vi "Gamma Noise.vi"(7 "initialize?":bool=TRUE, 9 "seed":i32=-1, 10 "order":i32=1, 11 "samples":i32=128) -> (0 "error":i32, 3 "gamma noise":dbl[](array[numeric]))   [LabVIEW 2020, in "NI_AALBase.lvlib"]
doc: "Generates a pseudorandom pattern of values that are the waiting times to the <B>order</B> number event of a unit mean Poisson process."
uses:
  <vilib>/Analysis/NI_AALBase.lvlib
  <resource>/lvanlys.dll
panel:
  # "Gamma Noise"
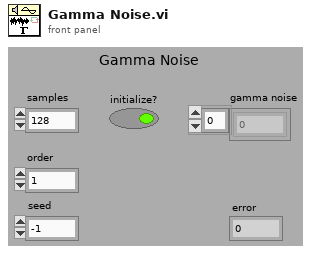
[diagram p1: front panel]
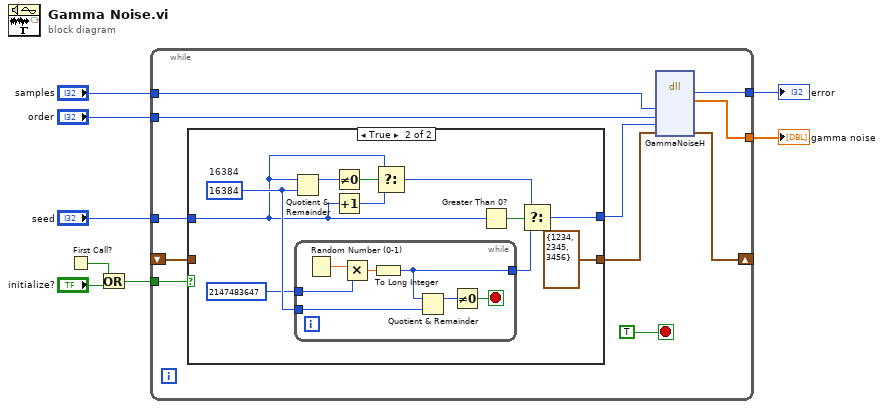
[diagram p0: block diagram]
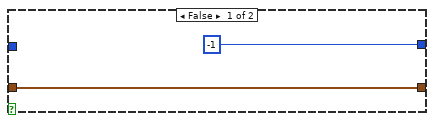
[diagram p2: hidden frame]
diagram:
  n1 = First Call?() -> (First Call?: T/F=w3:bool)
  n2 = Or(x=w3, y="initialize?") -> (x .or. y?=w1:bool)
  n3 = while {
    tunnel: [w16] -> w8
    tunnel: "seed" -> [w15]
    tunnel: "order" -> [w19]
    tunnel: "samples" -> [w18]
    shift-right: [w11] -> _
    shift-left: _ -> [w13]
    tunnel: w1 -> [w10]
    tunnel: [w9] -> w4
    stop <- TRUE stop-if-true
    n4 = case shown="True" w10 {
      tunnel: w13 -> [w21 _]
      tunnel: [w21 cluster{"xSeed":i32, "ySeed":i32, "zSeed":i32} {"xSeed"=1234, "ySeed"=2345, "zSeed"=3456} ("RNGState")] -> w12
      tunnel: [-1 ("seed") w22] -> w14
      tunnel: w15 -> [_ w23]
      frame False {
      }
      frame True {
        w25 = 16384  # 16384
        n5 = Quotient & Remainder(x=w23, y=w25) -> (x-y*floor(x/y)=w30:i32)  [unwired: 1 out]
        n6 = while {
          tunnel: [w37] -> w26
          tunnel: w25 -> [w36]
          tunnel: 2147483647 ("x") -> [w33]
          stop <- w34 stop-if-true
          n7 = Random Number (0-1)() -> (number: 0 to 1=w38:dbl)
          n8 = Multiply(x=w38, y=w33) -> (x*y=w39:dbl)
          n9 = To Long Integer(number=w39) -> (32bit integer=w37:i32)
          n10 = Quotient & Remainder(x=w37, y=w36) -> (x-y*floor(x/y)=w35:i32)  [unwired: 1 out]
          n11 = Not Equal To 0?(x=w35) -> (x != 0?=w34:bool)
        }
        n12 = Not Equal To 0?(x=w30) -> (x != 0?=w29:bool)
        n13 = Increment(x=w23) -> (x+1=w28:i32)
        n14 = Select(t=w23, s=w29, f=w28) -> (s? t:f=w27:i32)
        n15 = Greater Than 0?(x=w23) -> (x > 0?=w31:bool)
        n16 = Select(t=w27, s=w31, f=w26) -> (s? t:f=w22:i32)
      }
    }
    n17 = dll-call lib="e:/builds/penguin/labview/branches/2020/dev/dist/resource/lvanlys.*" fn="GammaNoiseH"("size"=w18, "order"=w19, "theSeed"=w14, "rngState"=w12) -> ("return type"=w16:i32, "xH"=w9:dbl[], "rngState"=w11:cluster{"xSeed":i32, "ySeed":i32, "zSeed":i32})  [unwired: 6 in, 3 out]
  }
  "error" <- w8
  "gamma noise" <- w4
